vi "Creators Status Created Events.vi"(11 "TEMPLATE Event in":refnum<class "TEMPLATE Event.lvclass">) -> (0 "Created Event Count":i32, 1 "Created Event Aliases":string[](array[string]), 2 "Created Event Exist?":bool, 3 "TEMPLATE Event out":refnum<class "TEMPLATE Event.lvclass">)   [LabVIEW 2021, in "_Template.lvlib" / "Templates.lvlib" / "TEM Event.lvlib" / "TEMPLATE Event.lvclass"]
uses:
  TEMPLATE Event.lvclass
  TEMPLATE Event.lvclass/TEMPLATE Event.ctl
  <vilib>/Nathan Davis/jettl/jettl/Event/Event.lvclass
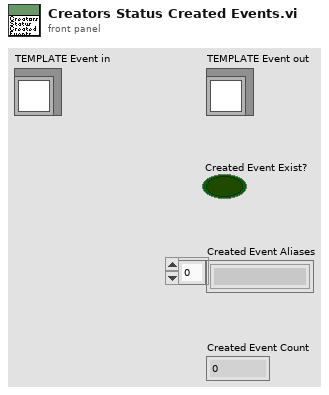
[diagram p1: front panel]
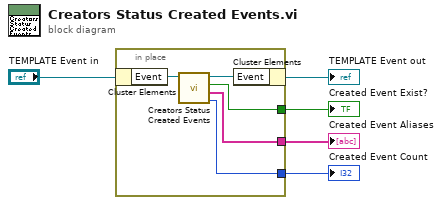
[diagram p0: block diagram]
diagram:
  n1 = in-place {
    in-place-border: [w8] -> w3
    in-place-border: [w7] -> w2
    in-place-border: [w6] -> w1
    n2 = in-place-cluster #1("TEMPLATE Event in") -> ("Event"=w10:refnum<class "Event.lvclass">)
    n3 = call-dynamic "Creators Status Created Events.vi"("Event in"=w10) -> ("Created Event Count"=w7:i32, "Created Event Aliases"=w6:string[], "Created Event Exist?"=w8:bool, "Event out"=w9:refnum<class "Event.lvclass">)  [unwired: 7 in]
    n4 = in-place-cluster #1("Event"=w9) -> (→"TEMPLATE Event out":refnum<class "TEMPLATE Event.lvclass">)
  }
  "Created Event Aliases" <- w1
  "Created Event Count" <- w2
  "Created Event Exist?" <- w3
